vi "Actor Core.vi"(8 "error in (no error)":errorcluster, 11 "Actor in":refnum<class "Tesla Tester GUI.lvclass">) -> (0 "error out":errorcluster, 3 "Actor out":refnum<class "Actor.lvclass">)   [LabVIEW 2013, in "Tesla Tester GUI.lvlib" / "Tesla Tester GUI.lvclass"]
uses:
  Tesla Tester GUI.lvclass
  <vilib>/ActorFramework/Actor/Actor.lvclass
  Tesla Factory Tester/Tesla Factory Tester_Actor/Tesla Factory Tester.lvclass/Tesla Factory Tester.ctl
  Tesla Tester GUI.lvclass/Tesla Tester GUI.ctl
  Tesla Factory Tester/Tesla Factory Tester_Actor/Tesla Factory Tester.lvclass
  <vilib>/ActorFramework/Actor/Actor.lvclass/Actor.ctl
  <vilib>/ActorFramework/Message Enqueuer/Message Enqueuer.lvclass/Message Enqueuer.ctl
  Ping Test/Ping Test_Actor/Ping Test.lvclass
  Text Based Test/Text Based Test_Actor/Text Based Test.lvclass
  CAN Protocol Test/CAN Protocol Test_Actor/CAN Protocol Test.lvclass
  Tesla Factory Tester/Messages/Run Tests_Msg/Run Tests_Msg.lvclass/Run Tests_Msg.ctl
  Tesla Factory Tester/Tesla Factory Tester_Actor/Write Status Str Refnum.vi
  <vilib>/ActorFramework/Message Enqueuer/Init from Existing Queue.vi
  <vilib>/ActorFramework/Message Enqueuer/Enqueue.vi
  <vilib>/ActorFramework/Message Priority Queue/Priority Enqueue.vi
  <vilib>/ActorFramework/Message Enqueuer/Message Enqueuer.lvclass
  <vilib>/ActorFramework/Stop Msg/Stop Msg.lvclass
  _test class base/_test class base_Actor/_test class base.lvclass
  Tesla Factory Tester/Messages/Run Tests_Msg/Run Tests_Msg.lvclass
panel:
  out "Status":string
  in  "Run tests":bool
  in  "List of tests":i32[](listbox) caption="Use standard windows/mac stuff here.  Hold 'control' button to select more than one test to run.\nAssuming touch screen, hence large buttons."
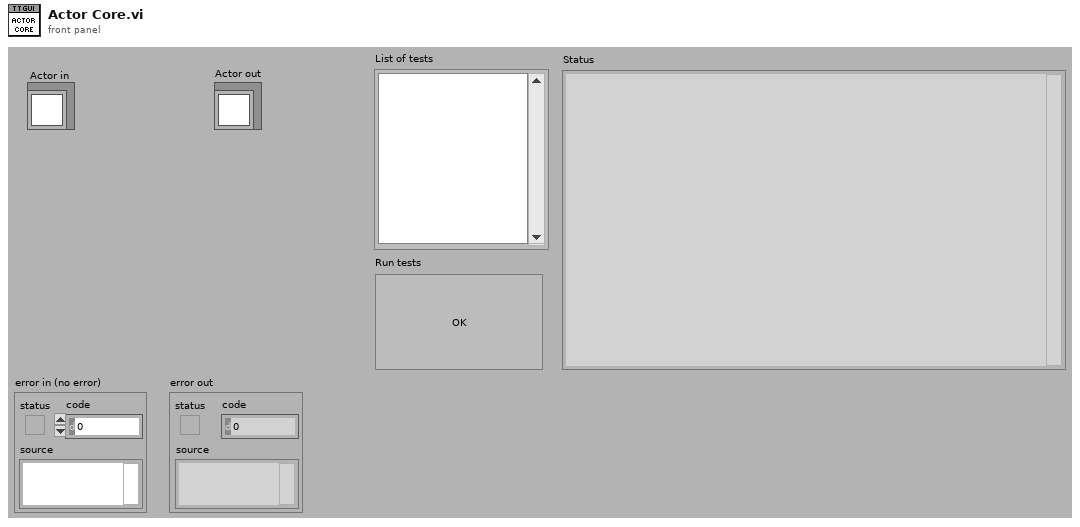
[diagram p1: front panel]
types:
  T1 = enum32{"invalid app kind", "Development System", "Run Time System", "Student Edition", "Embedded LabVIEW", "Evaluation", "Custom"}
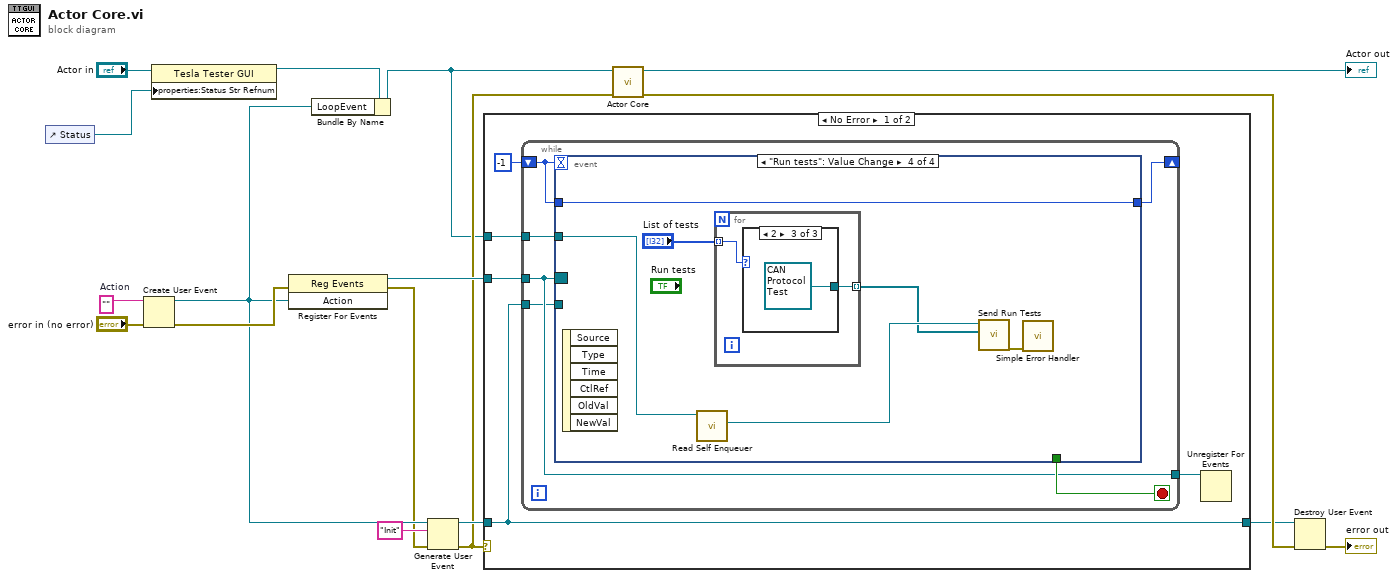
[diagram p0: block diagram]
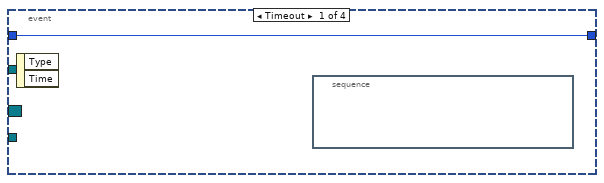
[diagram p2: hidden frame]
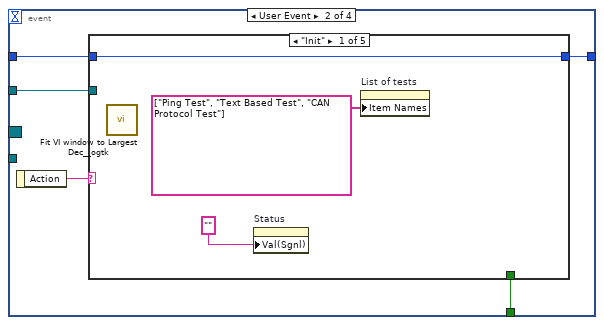
[diagram p3: hidden frame]
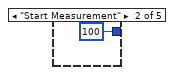
[diagram p4: hidden frame]
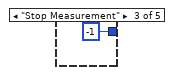
[diagram p5: hidden frame]
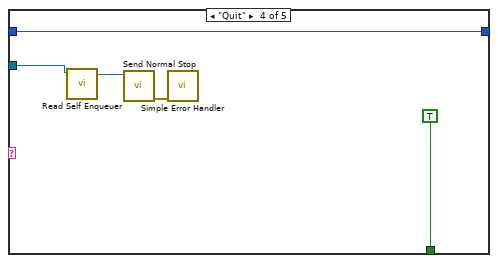
[diagram p6: hidden frame]
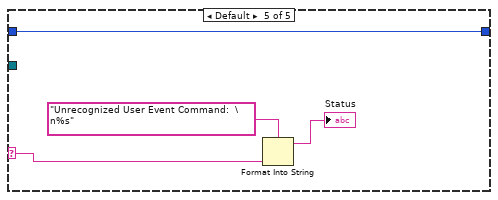
[diagram p7: hidden frame]
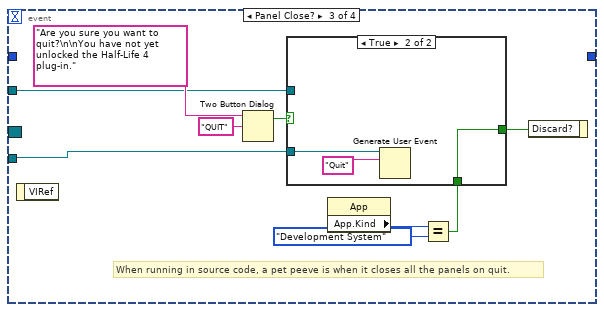
[diagram p8: hidden frame]
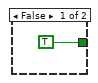
[diagram p9: hidden frame]
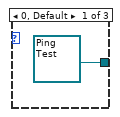
[diagram p10: hidden frame]
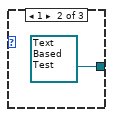
[diagram p11: hidden frame]
diagram:
  w14 = ""  # Action
  n1 = control-ref of="Status"() -> (w1:refnum<vi>)
  n2 = Create User Event(user event datatype=w14, error in="error in (no error)") -> (user event=w9:refnum<user-event>, error out=w15:errorcluster)
  n3 = property class="Tesla Tester GUI"(reference="Actor in", "properties:Status Str Refnum"=w1) -> (reference out=w2:refnum<class "Tesla Tester GUI.lvclass">)  [unwired: 1 in, 1 out]
  n4 = register-events(error in=w15, w9) -> (reference out=w16:refnum<event-registration>, error out=w5:errorcluster)  [unwired: 1 in]
  n5 = Bundle By Name(cluster=w2, "LoopEvent"=w9) -> (w4:refnum<class "Tesla Tester GUI.lvclass">)
  n6 = Generate User Event(user event=w9, event data cluster="Init" ("event data"), error in=w5) -> (user event out=w8:refnum<user-event>, error out=w7:errorcluster)  [unwired: 1 in]
  n7 = case shown="No Error" w7 {
    tunnel: w16 -> [w20 _]
    tunnel: [w19 w73] -> w10
    tunnel: w8 -> [w19 w73]
    tunnel: w4 -> [w18 _]
    frame No Error {
      n8 = while {
        shift-right: [w27] -> _
        shift-left: -1 -> [w28]
        tunnel: w20 -> [w25]
        tunnel: [w25] -> w21
        tunnel: w19 -> [w24]
        tunnel: w18 -> [w23]
        stop <- w26 stop-if-true
        n9 = event shown="[3] \"Run tests\": Value Change" {
          selector: w25 -> [_ _ _ _]
          dyn-events: _ -> [_ _ _ _]
          timeout: w28 -> [_ _ _ _]
          tunnel: w28 -> [w29 w33 _ w67]
          tunnel: [w29 w32 _ w67] -> w27
          tunnel: [_ w31 _ _] -> w26
          tunnel: w24 -> [_ _ w49 _]
          tunnel: w23 -> [_ w30 w52 w65]
          event Timeout {
            n10 = event-data() -> ()  [unwired: 1 in, 2 out]
            n11 = stacked-sequence {
              frame #0 {
              }
            }
          }
          event User Event {
            n12 = event-data() -> ("Action"=w34:string)  [unwired: 1 in]
            n13 = case shown="\"Init\"" w34 {
              selector: w34 -> [_ _ _ _ w46]
              tunnel: w33 -> [w37 _ _ w44 w48]
              tunnel: [w37 100 -1 w44 w48] -> w32
              tunnel: [_ _ _ TRUE _] -> w31
              tunnel: w30 -> [_ _ _ w40 _]
              frame "Init" {
                n14 = call <userlib>:"Fit VI window to Largest Dec__ogtk.vi"() -> ()  [unwired: 6 in, 2 out]
                n15 = property on="Status" class="Str"("Val(Sgnl)"="") -> ()  [unwired: 2 in, 2 out]
                n16 = property on="List of tests" class="LstBox (strict)"("Item Names"=string[] ["Ping Test", "Text Based Test", "CAN Protocol Test"]) -> ()  [unwired: 2 in, 2 out]
              }
              frame "Start Measurement" {
              }
              frame "Stop Measurement" {
              }
              frame "Quit" {
                n17 = call <vilib>:"Read Self Enqueuer.vi"("Actor"=w40) -> ("Self Enqueuer"=w42:refnum<class "Message Enqueuer.lvclass">)  [unwired: 10 in]
                n18 = call <vilib>:"Send Normal Stop.vi"("Message Enqueuer"=w42) -> ("error out"=w41:errorcluster)  [unwired: 10 in]
                n19 = call <vilib>:"Simple Error Handler.vi"("error in (no error)"=w41) -> ()  [unwired: 4 in, 5 out]
              }
              frame Default {
                n20 = Format Into String(format string="Unrecognized User Event Command:  \n%s", w46) -> (resulting string=→"Status":string)  [unwired: 2 in, 1 out]
              }
            }
          }
          event Panel Close? {
            # "When running in source code, a pet peeve is when it closes all the panels on quit."
            n21 = event-data() -> ()  [unwired: 1 in, 1 out]
            n22 = Two Button Dialog(message="Are you sure you want to quit?\n\nYou have not yet unlocked the Half-Life 4 plug-in.", 2:"QUIT" ("T button name (\"OK\")")) -> (T button?=w53:bool)  [unwired: 1 in]
            n23 = property class="App"() -> ("App.Kind"=w55:T1)  [unwired: 2 in, 2 out]
            n24 = Equal?(x=w55, y=T1."Development System") -> (x = y?=w50:bool)
            n25 = case shown="True" w53 {
              tunnel: w52 -> [_ _]
              tunnel: [TRUE w61] -> w51
              tunnel: w50 -> [_ w61]
              tunnel: w49 -> [_ w60]
              frame False {
              }
              frame True {
                n26 = Generate User Event(user event=w60, event data cluster="Quit" ("T button name (\"OK\")")) -> ()  [unwired: 2 in, 2 out]
              }
            }
            n27 = event-data("Discard?"=w51) -> ()  [unwired: 1 in, 1 out]
          }
          event "Run tests": Value Change {
            n28 = event-data() -> ()  [unwired: 1 in, 6 out]
            n29 = call <vilib>:"Read Self Enqueuer.vi"("Actor"=w65) -> ("Self Enqueuer"=w64:refnum<class "Message Enqueuer.lvclass">)  [unwired: 10 in]
            n30 = for {
              tunnel: "List of tests" -> [w68] mode=indexing
              tunnel: [w69] -> w63 mode=indexing
              n31 = case shown="2" w68 {
                tunnel: [refnum<class "Ping Test.lvclass"> refnum ("Ping Test.lvlib:Ping Test") refnum<class "Text Based Test.lvclass"> refnum ("Text Based Test.lvlib:Text Based Test") refnum<class "CAN Protocol Test.lvclass"> refnum ("CAN Protocol Test.lvlib:CAN Protocol Test")] -> w69
                frame 0, Default {
                }
                frame 1 {
                }
                frame 2 {
                }
              }
            }
            n32 = call "Send Run Tests.vi"("Tests to Run"=w63, "Message Enqueuer"=w64) -> ("error out"=w62:errorcluster)  [unwired: 8 in, 1 out]
            n33 = call <vilib>:"Simple Error Handler.vi"("error in (no error)"=w62) -> ()  [unwired: 4 in, 5 out]
          }
        }
      }
      n34 = Unregister For Events(event registration refnum=w21) -> ()  [unwired: 1 in, 1 out]
    }
    frame Error {
    }
  }
  n35 = call-parent "Actor Core.vi"("error in"=w7, "Actor in"=w4) -> ("error out"=w11:errorcluster, "Actor out"=→"Actor out":refnum<class "Actor.lvclass">)  [unwired: 8 in]
  n36 = Destroy User Event(user event=w10, error in=w11) -> (error out=→"error out":errorcluster)
